vi "Telnet Read Filter.vi"(4 "error in":errorcluster, 5 "unfiltered data in":string, 7 "Connection in":refnum<k5>) -> (0 "error out":errorcluster, 1 "Unfiltered data out":string, 2 "Data out":string, 3 "connection out":refnum<k5>)   [LabVIEW 2015, in "NI_InternetTK_Core_VIs.lvlib"]
uses:
  NI_InternetTK_Core_VIs.lvlib
  NI_InternetTK_Common_VIs.lvlib
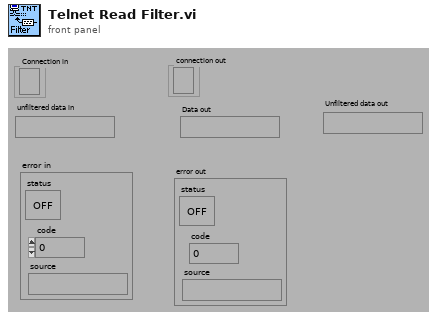
[diagram p1: front panel]
types:
  T1 = cluster{"command":enum16{"WILL", "WON'T", "DO", "DON'T"}, "option":u8}
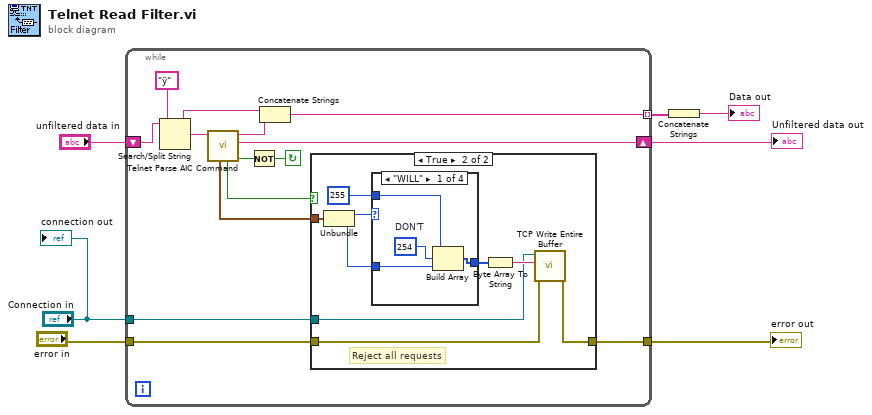
[diagram p0: block diagram]
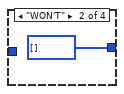
[diagram p3: hidden frame]
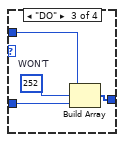
[diagram p4: hidden frame]
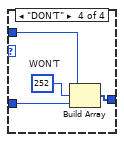
[diagram p5: hidden frame]
diagram:
  n1 = while {
    tunnel: [w8] -> w2 mode=indexing
    tunnel: [w10] -> w5
    tunnel: "Connection in" -> [w9]
    tunnel: "error in" -> [w11]
    shift-left: "unfiltered data in" -> [w20]
    shift-right: [w18] -> w3
    stop <- w14 continue-if-true
    n2 = Search/Split String(string=w20, search string/char (-)="ÿ" ("regular expression")) -> (substring before match=w17:string, match + rest of string=w19:string)  [unwired: 2 out]
    n3 = call "Telnet Parse AIC Command.vi"("AIC sequence"=w19) -> ("error"=w15:bool, "after sequence"=w18:string, "AIC result"=w16:string, "option negotiation"=w13:bool, "option info"=w12:T1)  [unwired: 6 out]
    n4 = Not(x=w15) -> (.not. x?=w14:bool)
    n5 = Concatenate Strings(w17, w16) -> (w8:string)
    n6 = case shown="True" w13 {
      tunnel: w12 -> [_ w31]
      tunnel: w11 -> [w22 w26]
      tunnel: [w22 w25] -> w10
      tunnel: w9 -> [_ w24]
      frame False {
      }
      frame True {
        # "Reject all requests"
        n7 = Unbundle(w31) -> ("command"=w30:enum16{"WILL", "WON'T", "DO", "DON'T"}, "option"=w29:u8)
        n8 = case shown="\"WILL\"" w30 {
          tunnel: w29 -> [w35 _ w40 w44]
          tunnel: [w33 u8[] [] w38 w42] -> w28
          tunnel: u8 255 -> [w32 _ w37 w41]
          frame "WILL" {
            w34 = u8 254  # DON'T
            n9 = Build Array(w32, w34, w35) -> (w33:u8[])
          }
          frame "WON'T" {
          }
          frame "DO" {
            w39 = u8 252  # WON'T
            n10 = Build Array(w37, w39, w40) -> (w38:u8[])
          }
          frame "DON'T" {
            w43 = u8 252  # WON'T
            n11 = Build Array(w41, w43, w44) -> (w42:u8[])
          }
        }
        n12 = Byte Array To String(unsigned byte array=w28) -> (string=w27:string)
        n13 = call "TCP Write Entire Buffer.vi"("error in (no error)"=w26, "data in"=w27, "connection ID"=w24) -> ("error out"=w25:errorcluster)  [unwired: 8 out]
      }
    }
  }
  "Unfiltered data out" <- w3
  "error out" <- w5
  n14 = Concatenate Strings(w2) -> (→"Data out":string)
  "connection out" <- "Connection in"
